vi "Is Error.vi"(11 "jettl Queue Actor in":refnum<class "jettl Queue Actor.lvclass">) -> (3 "jettl Queue Actor out":refnum<class "jettl Queue Actor.lvclass">)   [LabVIEW 2021, in "jettl Queue Actor.lvlib" / "jettl Queue Actor.lvclass"]
uses:
  jettl Queue Actor.lvclass
  State/Nominal State/Nominal State.lvclass
  C:/git/jettl/src/jettl/jettl Queue Actor/State/State/State.lvclass
  State/Error State/Error State.lvclass
  jettl Queue Actor.lvclass/jettl Queue Actor.ctl
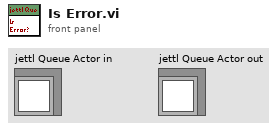
[diagram p1: front panel]
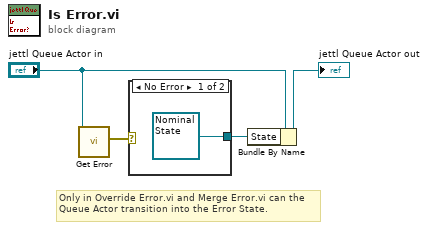
[diagram p0: block diagram]
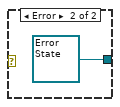
[diagram p2: hidden frame]
diagram:
  # "Only in Override Error.vi and Merge Error.vi can the Queue Actor transition into the Error State."
  n1 = call-dynamic "Get Error.vi"("jettl Queue Actor in"="jettl Queue Actor in") -> ("Error"=w4:errorcluster)  [unwired: 10 in]
  n2 = case shown="No Error" w4 {
    tunnel: [refnum<class "Nominal State.lvclass"> refnum ("jettl.lvlib:jettl Queue Actor.lvlib:Nominal State.lvclass") refnum<class "Error State.lvclass"> refnum ("jettl.lvlib:jettl Queue Actor.lvlib:Error State.lvclass")] -> w1
    frame No Error {
    }
    frame Error {
    }
  }
  n3 = Bundle By Name(cluster="jettl Queue Actor in", "State"=w1) -> (→"jettl Queue Actor out":refnum<class "jettl Queue Actor.lvclass">)
